vi "Get Microscope Image.vi"() -> ()   [LabVIEW 2014]
uses:
  <vilib>/vision/Avi1.llb/AviRefnum.ctl
panel:
  in  "Capture Video":bool
  in  "Video Index":dbl=1.0 min=1.0 step=1.0
  in  "New Video File":bool
  in  "Reset Averaging":bool
  in  "Averaging":bool
  in  "Image Index":dbl
  in  "Capture and Save Image":bool
  in  "path to save files":path
  in  "stop":bool
  out "Image":u32[][](graph)
  out "used request":i32
  in  "Video channel":i32=3
  # "Must use stop button to abort or else video driver screwed up!"
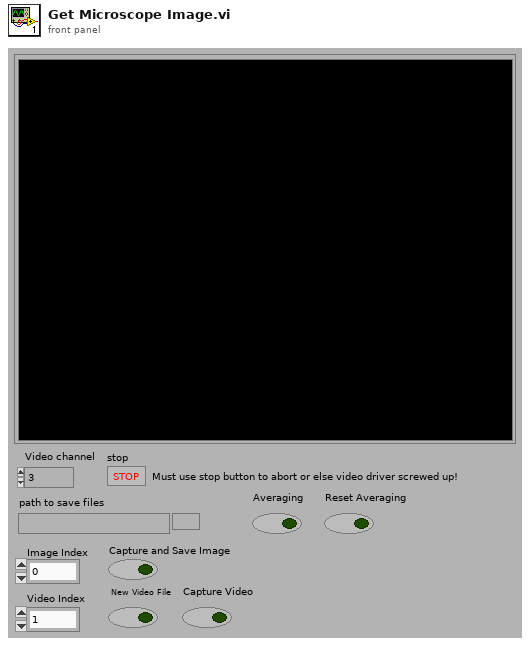
[diagram p1: front panel]
types:
  T1 = enum32{"setting", "request", "request control", "info", "statistics", "system settings", "I/O sub system", "HRT control", "camera descriptions", "device specific data", "event sub system settings", "event sub system results", "image memory manager"}
  T2 = typedef "AviRefnum.ctl" = refnum<k1>
  T3 = typedef "Image Type" = u32
  T4 = typedef "IMAQ Image.ctl" = refnum<image>
  T5 = typedef "imagedata.ctl" = cluster{"image type":i32, "image depth":i32, "image":u8[], "mask":u8[], "colors":u32[], "Rectangle":cluster{"left":i16, "top":i16, "right":i16, "bottom":i16}}
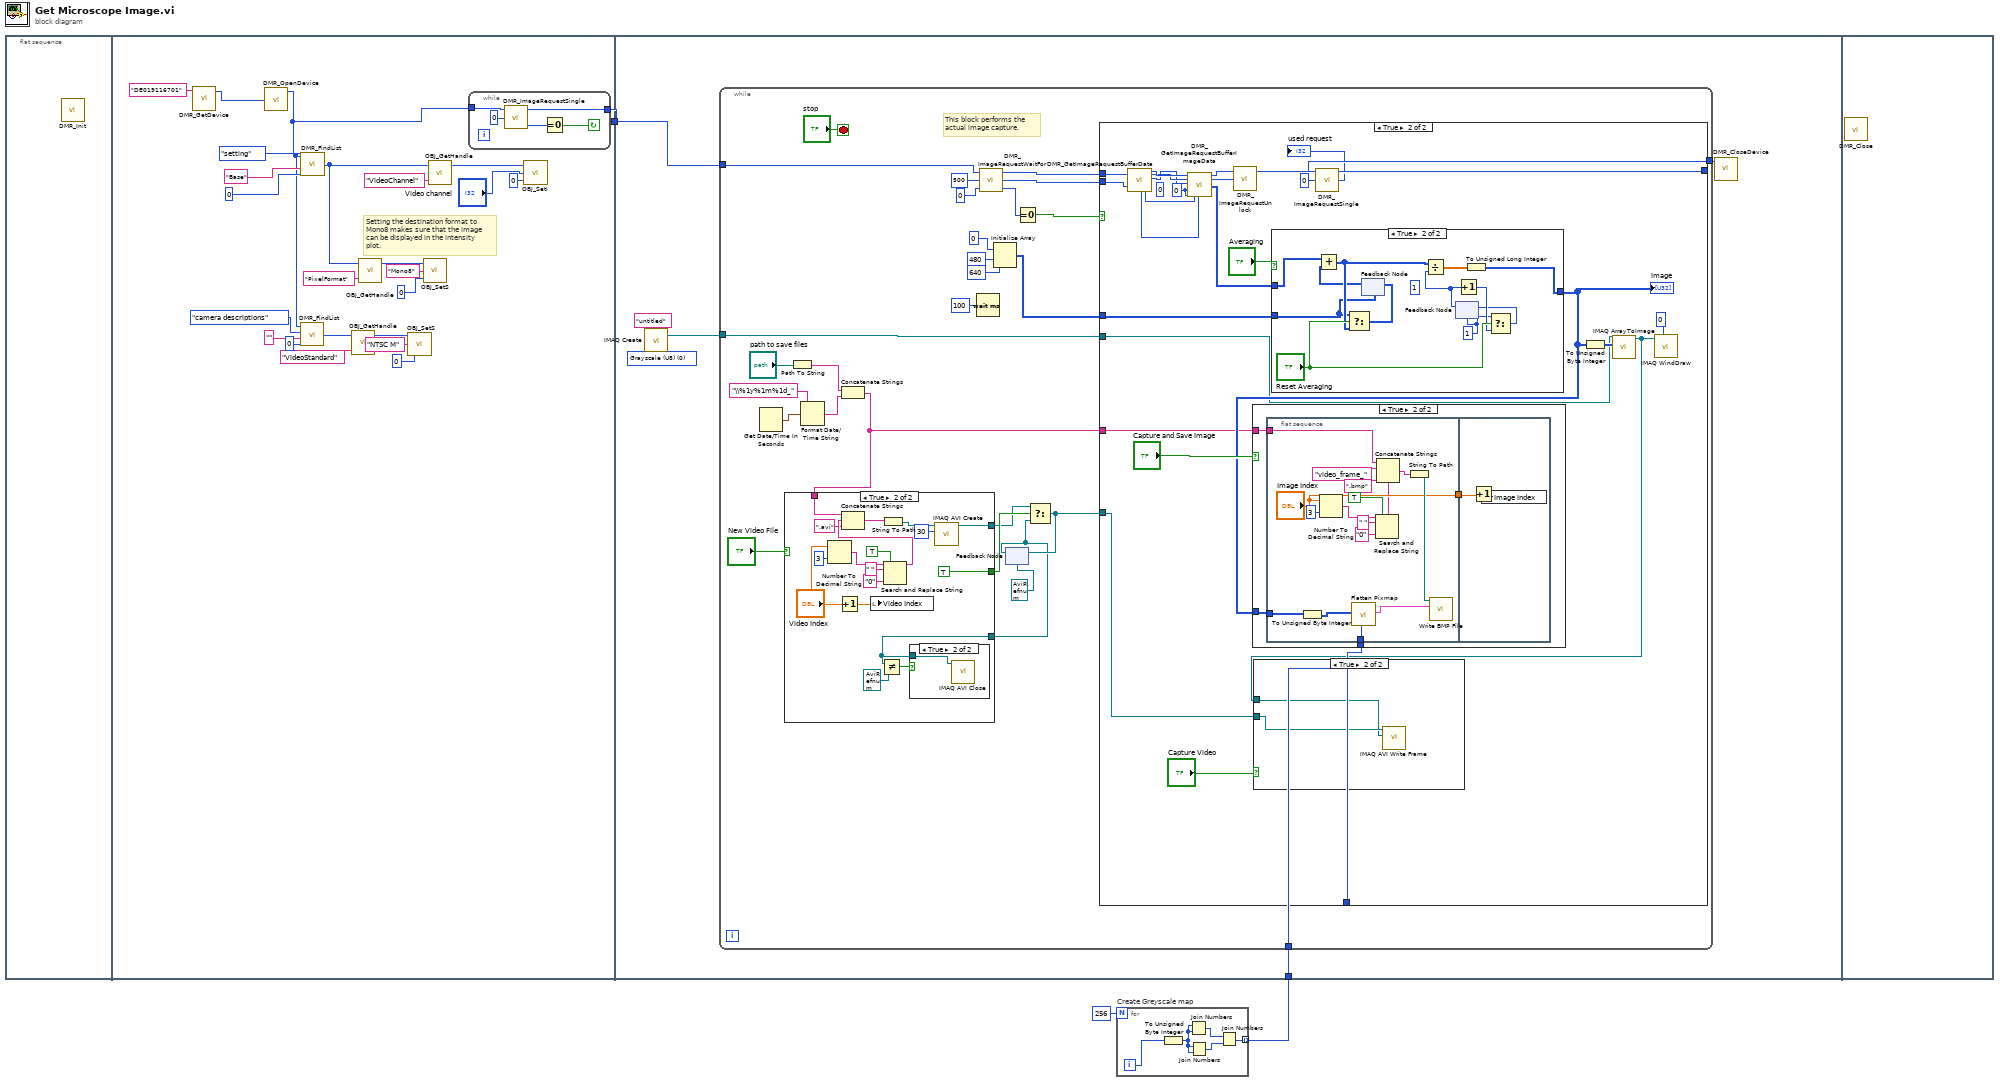
[diagram p0: block diagram]
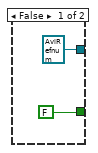
[diagram p2: hidden frame]
diagram:
  n1 = flat-sequence {
    tunnel: [w8] -> w3
    tunnel: w3 -> [w38]
    tunnel: w1 -> [w36]
    frame #0 {
      n2 = call "DMR_Init.vi"() -> ()  [unwired: 1 in, 2 out]
    }
    frame #1 {
      # "Setting the destination format to Mono8 makes sure that the image can be displayed in the intensity plot."
      n3 = call "DMR_GetDevice.vi"("search string IN"="DE019116701") -> ("device handle OUT"=w26:i32)  [unwired: 5 in, 1 out]
      n4 = call "DMR_OpenDevice.vi"("device handle IN"=w26) -> ("driver handle OUT"=w9:i32)  [unwired: 2 in, 2 out]
      n5 = call "DMR_FindList.vi"("flags IN"=u32 0 ("flags"), "list name IN"="" ("String"), "list type IN"=T1."camera descriptions", "driver handle IN"=w9) -> ("list handle OUT"=w12:i32)  [unwired: 2 out]
      n6 = call "DMR_FindList.vi"("flags IN"=u32 0 ("flags"), "list name IN"="Base", "list type IN"=T1."setting", "driver handle IN"=w9) -> ("list handle OUT"=w10:i32)  [unwired: 2 out]
      n7 = call "OBJ_GetHandle.vi"("object name IN"="VideoStandard", "list handle IN"=w12) -> ("object handle OUT"=w6:i32)  [unwired: 2 in, 1 out]
      n8 = call "OBJ_GetHandle.vi"("object name IN"="PixelFormat", "list handle IN"=w10) -> ("object handle OUT"=w20:i32)  [unwired: 2 in, 1 out]
      n9 = call "OBJ_SetS.vi"("value index IN"=0, "value IN"="NTSC M", "object handle IN"=w6) -> ()  [unwired: 2 out]
      n10 = call "OBJ_SetS.vi"("value index IN"=0, "value IN"="Mono8" ("value"), "object handle IN"=w20) -> ()  [unwired: 2 out]
      n11 = call "OBJ_GetHandle.vi"("object name IN"="VideoChannel", "list handle IN"=w10) -> ("object handle OUT"=w16:i32)  [unwired: 2 in, 1 out]
      n12 = while {
        tunnel: [w31] -> w8
        tunnel: w9 -> [w28]
        stop <- w29 continue-if-true
        n13 = call "DMR_ImageRequestSingle.vi"("request control IN"=0, "driver handle IN"=w28) -> ("error code OUT"=w30:i32, "driver handle OUT"=w31:i32)  [unwired: 1 in, 1 out]
        n14 = Equal To 0?(x=w30) -> (x = 0?=w29:bool)
      }
      n15 = call "OBJ_SetI.vi"("value index IN"=0, "value IN"="Video channel", "object handle IN"=w16) -> ()  [unwired: 2 out]
    }
    frame #2 {
      w33 = T3 0 items=["Grayscale (U8)", "Grayscale (I16)", "Grayscale (SGL)", "Complex (CSG)", "RGB (U32)", "HSL (U32)", "RGB (U64)"] ("Image Type")
      n16 = call "IMAQ Create"("Image Name"="untitled", "Image Type"=w33) -> ("New Image"=w34:T4)  [unwired: 3 in, 1 out]
      n17 = while {
        tunnel: w38 -> [w60]
        tunnel: [w59] -> w37
        tunnel: w36 -> [w56]
        tunnel: w34 -> [w55]
        stop <- "stop" stop-if-true
        # "This block performs the \nactual image capture."
        n18 = Get Date/Time In Seconds() -> (seconds since 1Jan1904=w47:timestamp)
        n19 = Path To String(path="path to save files") -> (string=w50:string)
        n20 = Format Date/Time String(time format string (%c)="\\%1y%1m%1d_", seconds (now)=w47) -> (date/time string=w49:string)  [unwired: 1 in]
        n21 = Concatenate Strings(w50, w49) -> (w44:string)
        n22 = Wait (ms)(milliseconds to wait=u32 100) -> ()  [unwired: 1 out]
        n23 = call "DMR_ImageRequestWaitFor.vi"("queue number IN"=0, "timeout(ms) IN"=500, "driver handle IN"=w60) -> ("error code OUT"=w64:i32, "request number OUT"=w61:i32, "driver handle OUT"=w62:i32)
        n24 = Initialize Array(u32 0 ("Window Number (0...15)"), 480 ("dimension size"), 640 ("dimension size")) -> (w51:u32[][])
        n25 = feedback #1(T2 refnum ("Avi Refnum")) -> (w39:T2)
        n26 = case shown="True" "New Video File" {
          tunnel: w44 -> [_ w86]
          tunnel: [T2 refnum ("Avi Refnum") w73] -> w41
          tunnel: [FALSE TRUE] -> w42
          tunnel: w39 -> [_ w69]
          frame False {
          }
          frame True {
            n27 = Number To Decimal String(number="Video Index", width (-)=i16 3) -> (decimal integer string=w80:string)
            n28 = Increment(x="Video Index") -> (x+1=w85:dbl)
            n29 = local write "Video Index"(w85) -> ()
            n30 = Not Equal?(x=w69, y=T2 refnum ("Avi Refnum")) -> (x != y?=w70:bool)
            n31 = Search and Replace String(replace all?=TRUE ("replace all? (F)"), input string=w80, search string=" ", replace string="0" ("replace string (\"\")")) -> (result string=w78:string)  [unwired: 4 in, 3 out]
            n32 = Concatenate Strings(w86, w78, ".avi" ("string")) -> (w76:string)
            n33 = String To Path(string=w76) -> (path=w75:path)
            n34 = case shown="True" w70 {
              tunnel: w69 -> [_ w87]
              frame False {
              }
              frame True {
                n35 = call "IMAQ AVI Close"("Avi Refnum"=w87) -> ()  [unwired: 10 in, 1 out]
              }
            }
            n36 = call "IMAQ AVI Create"("Frames Per Second"=u32 30, "AVI Path"=w75) -> ("Avi Refnum"=w73:T2)  [unwired: 8 in, 1 out]
          }
        }
        n37 = Equal To 0?(x=w64) -> (x = 0?=w63:bool)
        n38 = Select(t=w41, s=w42, f=w39) -> (s? t:f=w40:T2)
        n39 = feedback-in #1(w40) -> ()
        n40 = case shown="True" w63 {
          tunnel: w62 -> [w88 w115]
          tunnel: w61 -> [_ w114]
          tunnel: [w88 w111] -> w59
          tunnel: w56 -> [_ w100]
          tunnel: w55 -> [_ w93]
          tunnel: w51 -> [_ w96]
          tunnel: w44 -> [_ w92]
          tunnel: w40 -> [_ w90]
          frame False {
          }
          frame True {
            w104 = u32 0 ("X-offset IN")
            (unwired) u32 0 ("X-offset")
            n41 = call "DMR_GetImageRequestBufferData.vi"("driver handle IN"=w115, "request number IN"=w114) -> ("width OUT"=w103:i32, "height OUT"=w102:i32, "driver handle OUT"=w109:i32, "request number OUT"=w108:i32, "bytes per pixel OUT"=w105:i32)  [unwired: 8 in, 5 out]
            n42 = call "DMR_GetImageRequestBufferImageData.vi"("driver handle IN"=w109, "request number IN"=w108, "bytes per pixel IN"=w105, "X-offset IN"=w104, "Y-offset IN"=w104, "height IN"=w102, "width IN"=w103) -> ("driver handle OUT"=w107:u32, "request number OUT"=w106:u32, "image OUT"=w97:u32[][])  [unwired: 9 in, 1 out]
            n43 = call "DMR_ImageRequestUnlock.vi"("request number IN"=w106, "driver handle IN"=w107) -> ("driver handle OUT"=w113:i32)  [unwired: 2 in, 1 out]
            n44 = case shown="True" "Averaging" {
              tunnel: w97 -> [w118 w123]
              tunnel: [w118 w122] -> w94
              tunnel: w96 -> [_ w120]
              frame False {
              }
              frame True {
                (unwired) 1
                w128 = 1
                n45 = feedback #2(w120) -> (w119:u32[][])
                n46 = Add(x=w123, y=w119) -> (x+y=w124:u32[][])
                n47 = Select(t=w120, s="Reset Averaging", f=w124) -> (s? t:f=w126:u32[][])
                n48 = feedback-in #2(w126) -> ()
                n49 = feedback #3(w128) -> (w121:i32)
                n50 = Divide(x=w124, y=w121) -> (x/y=w125:dbl[][])
                n51 = Increment(x=w121) -> (x+1=w129:i32)
                n52 = To Unsigned Long Integer(number=w125) -> (unsigned 32bit integer=w122:u32[][])
                n53 = Select(t=w128, s="Reset Averaging", f=w129) -> (s? t:f=w127:i32)
                n54 = feedback-in #3(w127) -> ()
              }
            }
            "Image" <- w94
            n55 = case shown="True" "Capture and Save Image" {
              tunnel: w94 -> [_ w134]
              tunnel: w100 -> [_ w132]
              tunnel: w92 -> [_ w131]
              frame False {
              }
              frame True {
                n56 = flat-sequence {
                  tunnel: w134 -> [w143]
                  tunnel: ["Image Index"] -> w133
                  tunnel: w132 -> [w141]
                  tunnel: w131 -> [w135]
                  tunnel: w133 -> [w152]
                  frame #0 {
                    n57 = To Unsigned Byte Integer(number=w143) -> (unsigned 8bit integer=w142:u8[][])
                    n58 = Number To Decimal String(number="Image Index", width (-)=i16 3) -> (decimal integer string=w137:string)
                    n59 = call <vilib>:"Flatten Pixmap.vi"("colors"=w141, "8-bit pixmap"=w142) -> ("image data"=w150:T5)  [unwired: 9 in]
                    n60 = Search and Replace String(replace all?=TRUE ("replace all? (F)"), input string=w137, search string=" ", replace string="0" ("replace string (\"\")")) -> (result string=w136:string)  [unwired: 4 in, 3 out]
                    n61 = Concatenate Strings(w135, "video_frame_" ("string"), w136, ".bmp" ("string")) -> (w147:string)
                    n62 = String To Path(string=w147) -> (path=w146:path)
                    n63 = call <vilib>:"Write BMP File.vi"("image data"=w150, "path to BMP file"=w146) -> ()  [unwired: 8 in, 2 out]
                  }
                  frame #1 {
                    n64 = Increment(x=w152) -> (x+1=w151:dbl)
                    n65 = local write "Image Index"(w151) -> ()
                  }
                }
              }
            }
            n66 = call "DMR_ImageRequestSingle.vi"("request control IN"=0, "driver handle IN"=w113) -> ("request used OUT"=→"used request":i32, "driver handle OUT"=w111:i32)  [unwired: 1 in, 1 out]
            n67 = To Unsigned Byte Integer(number=w94) -> (unsigned 8bit integer=w95:u8[][])
            n68 = call "IMAQ ArrayToImage"("Image Pixels (U8)"=w95, "Image"=w93) -> ("Image Out"=w89:T4)  [unwired: 8 in, 1 out]
            n69 = case shown="True" "Capture Video" {
              tunnel: w90 -> [_ w117]
              tunnel: w89 -> [_ w116]
              frame False {
              }
              frame True {
                n70 = call "IMAQ AVI Write Frame"("Image"=w116, "Avi Refnum"=w117) -> ()  [unwired: 8 in, 2 out]
              }
            }
            n71 = call "IMAQ WindDraw"("Window Number (0...15)"=0, "Image"=w89) -> ()  [unwired: 8 in, 2 out]
          }
        }
      }
      n72 = call "DMR_CloseDevice.vi"("driver handle IN"=w37) -> ()  [unwired: 3 in, 2 out]
    }
    frame #3 {
      n73 = call "DMR_Close.vi"() -> ()  [unwired: 1 out]
    }
  }
  n74 = for "Create Greyscale map" {
    N: 256 -> [_]
    tunnel: [w154] -> w1 mode=indexing
    i -> [w157]
    n75 = To Unsigned Byte Integer(number=w157) -> (unsigned 8bit integer=w153:u8)
    n76 = Join Numbers(hi=w153, lo=w153) -> ((hi.lo)=w156:u16)
    n77 = Join Numbers(hi=w153, lo=w153) -> ((hi.lo)=w155:u16)
    n78 = Join Numbers(hi=w156, lo=w155) -> ((hi.lo)=w154:u32)
  }
